vi "Uneven.vi"(0 "number in":i32) -> (4 "uneven number out":i32)   [LabVIEW 2016]
doc: "Always returns an uneven number."
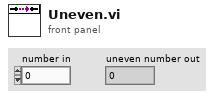
[diagram p1: front panel]
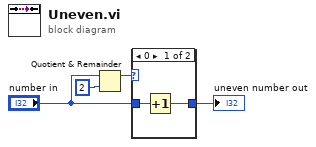
[diagram p0: block diagram]
diagram:
  n1 = Quotient & Remainder(x="number in", y=2) -> (x-y*floor(x/y)=w2:i32)  [unwired: 1 out]
  n2 = case shown="0" w2 {
    tunnel: [w5 w7] -> w4
    tunnel: "number in" -> [w6 w7]
    frame 0 {
      n3 = Increment(x=w6) -> (x+1=w5:i32)
    }
    frame 1, Default {
    }
  }
  "uneven number out" <- w4
